vi "ziOpen.vi"(3 "Error In":errorcluster, 4 "Port obsolete (auto)":u16, 5 "Hostname obsolete (auto)":string, 6 "Address":string="DEV") -> (0 "Error Out":errorcluster, 1 "Selected Device":string, 2 "HandleOut":T1 {"Handle" format="0x%08x"; "Conn" format="0x%08x"})   [LabVIEW 2019, in "Zurich Instruments LabOne.lvlib"]
doc: "Creates a connection to a Data Server. <b>Address</b> is of the format {<host>}{:<port}{::<Device ID>}. Usually it is sufficient to provide the <b>Device ID</b> only. The host and port are then determined by network discovery. Should the discovery not work, prepend <host>:<port>:: to the Device ID. Examples are \"myhf2.company.com:8004::dev466\" or \"myhf2.company.com:8004\". In the latter case the first found instrument on the data server listening on myhf2.company.com:8004 will be selected."
uses:
  Zurich Instruments LabOne.lvlib
  ziTypeHandle.ctl
  ziTypeDisovery.ctl
  Private/ziLV64.dll
panel:
  out "auto-connected":bool
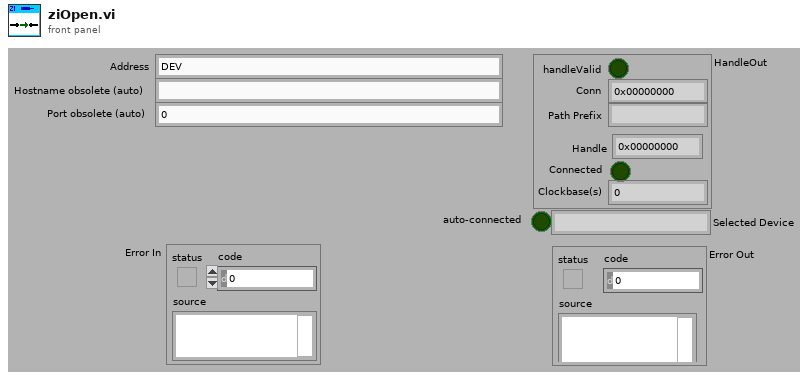
[diagram p1: front panel]
types:
  T1 = typedef "Zurich Instruments LabOne.lvlib/ziTypeHandle.ctl" = cluster{"handleValid":bool, "Conn":u64, "Path Prefix":string, "Handle":u64, "Connected":bool, "Clockbase(s)":dbl}
  T2 = typedef "Zurich Instruments LabOne.lvlib/ziTypeDisovery.ctl" = cluster{"timestamp":u64, "deviceid":string, "devicetype":string, "serveraddress":string, "serverport":u32, "apilevel":u32, "discoverable":bool, "interface":string, "connected":string, "available":bool, "owner":string, "status":string, "options ":string, "serverversion":string}
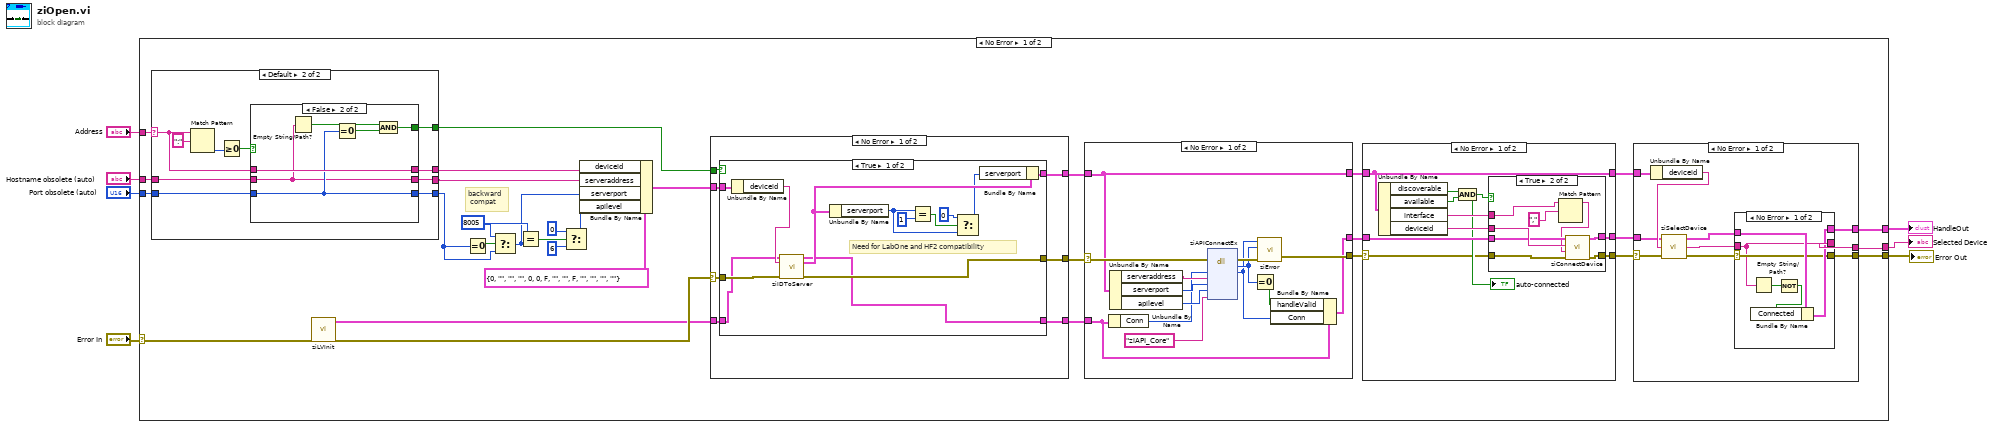
[diagram p0: block diagram]
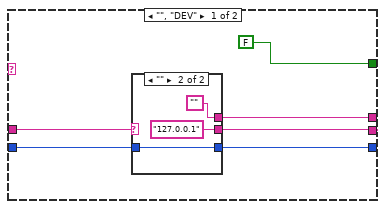
[diagram p2: hidden frame]
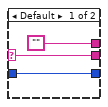
[diagram p3: hidden frame]
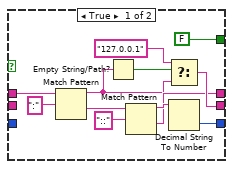
[diagram p4: hidden frame]
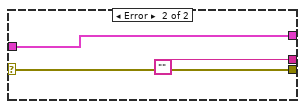
[diagram p6: hidden frame]
diagram:
  n1 = case shown="No Error" "Error In" {
    selector: "Error In" -> [w10 w167]
    tunnel: [w38 w167] -> w7
    tunnel: [w37 _] -> w6
    tunnel: "Hostname obsolete (auto)" -> [w30 _]
    tunnel: "Port obsolete (auto)" -> [w31 _]
    tunnel: [w36 _] -> w5
    tunnel: "Address" -> [w29 _]
    frame No Error {
      w16 = u32 8005
      # "backward\n compat"
      n2 = case shown="Default" w29 {
        selector: w29 -> [_ w53]
        tunnel: w30 -> [w44 w59]
        tunnel: w31 -> [w43 w55]
        tunnel: [w42 w60] -> w17
        tunnel: [w41 w58] -> w23
        tunnel: [w40 w57] -> w22
        tunnel: [FALSE w56] -> w19
        frame "", "DEV" {
          n3 = case shown="\"\"" w44 {
            selector: w44 -> [w46 _]
            tunnel: w43 -> [w45 w50]
            tunnel: [w45 w50] -> w42
            tunnel: [w46 "127.0.0.1"] -> w41
            tunnel: ["" ""] -> w40
            frame Default {
            }
            frame "" {
            }
          }
        }
        frame Default {
          n4 = Match Pattern(string=w53, regular expression=":") -> (offset past match=w54:i32)  [unwired: 1 in, 3 out]
          n5 = Greater Or Equal To 0?(x=w54) -> (x >= 0?=w51:bool)
          n6 = case shown="False" w51 {
            tunnel: [w65 w77] -> w60
            tunnel: w59 -> [_ w74]
            tunnel: [w67 w74] -> w58
            tunnel: w53 -> [w71 w78]
            tunnel: [w64 w78] -> w57
            tunnel: [FALSE w75] -> w56
            tunnel: w55 -> [_ w77]
            frame True {
              n7 = Match Pattern(string=w71, regular expression=":") -> (before substring=w62:string, after substring=w68:string)  [unwired: 1 in, 2 out]
              n8 = Empty String/Path?(string/path=w62) -> (empty?=w61:bool)
              n9 = Match Pattern(string=w68, regular expression="::") -> (before substring=w66:string, after substring=w64:string)  [unwired: 1 in, 2 out]
              n10 = Select(t="127.0.0.1", s=w61, f=w62) -> (s? t:f=w67:string)
              n11 = Decimal String To Number(string=w66) -> (number=w65:i32)  [unwired: 2 in, 1 out]
            }
            frame False {
              n12 = Empty String/Path?(string/path=w74) -> (empty?=w73:bool)
              n13 = Equal To 0?(x=w77) -> (x = 0?=w76:bool)
              n14 = And(x=w73, y=w76) -> (x .and. y?=w75:bool)
            }
          }
        }
      }
      n15 = call "ziLVInit.vi"("Error In"=w10) -> ("Error Out"=w9:errorcluster, "ziHandle"=w8:T1)  [unwired: 9 in]
      n16 = Equal To 0?(x=w17) -> (x = 0?=w18:bool)
      n17 = Select(t=w16, s=w18, f=w17) -> (s? t:f=w11:u32)
      n18 = Equal?(x=w16, y=w11) -> (x = y?=w15:bool)
      n19 = Select(t=u32 0, s=w15, f=u32 6) -> (s? t:f=w12:u32)
      n20 = Bundle By Name(cluster=T2 {"timestamp"=0, "deviceid"="", "devicetype"="", "serveraddress"="", "serverport"=0, "apilevel"=0, "discoverable"=FALSE, "interface"="", "connected"="", "available"=FALSE, "owner"="", "status"="", "options "="", "serverversion"=""} ("ziDiscovery"), "deviceid"=w22, "serveraddress"=w23, "serverport"=w11, "apilevel"=w12) -> (w25:T2)
      n21 = case shown="No Error" w9 {
        selector: w9 -> [w130 w149]
        tunnel: [w129 w149] -> w32
        tunnel: [w128 w147] -> w28
        tunnel: w19 -> [w127 _]
        tunnel: w25 -> [w126 w147]
        tunnel: w8 -> [w125 w148]
        tunnel: [w124 w148] -> w21
        frame No Error {
          n22 = case shown="True" w127 {
            tunnel: w130 -> [w143 w146]
            tunnel: [w142 w146] -> w129
            tunnel: [w140 w145] -> w128
            tunnel: w126 -> [w134 w145]
            tunnel: w125 -> [w131 w144]
            tunnel: [w132 w144] -> w124
            frame True {
              # "Need for LabOne and HF2 compatibility"
              n23 = Unbundle By Name(w134) -> ("deviceid"=w133:string)
              n24 = call "ziIDToServer.vi"("ziHandle In"=w131, "Device ID"=w133, "Error In"=w143) -> ("ziHandle Out"=w132:T1, "ziDiscovery"=w141:T2, "Error Out"=w142:errorcluster)  [unwired: 10 in]
              n25 = Unbundle By Name(w141) -> ("serverport"=w136:u32)
              n26 = Equal?(x=w136, y=u32 1) -> (x = y?=w138:bool)
              n27 = Select(t=u32 0, s=w138, f=w136) -> (s? t:f=w135:u32)
              n28 = Bundle By Name(cluster=w141, "serverport"=w135) -> (w140:T2)
            }
            frame False {
            }
          }
        }
        frame Error {
        }
      }
      n29 = case shown="No Error" w32 {
        selector: w32 -> [w159 w166]
        tunnel: [w162 w166] -> w33
        tunnel: w28 -> [w156 w165]
        tunnel: [w156 w165] -> w27
        tunnel: w21 -> [w152 w164]
        tunnel: [w151 w164] -> w20
        frame No Error {
          n30 = Unbundle By Name(w152) -> ("Conn"=w154:u64)
          n31 = Unbundle By Name(w156) -> ("serveraddress"=w158:string, "serverport"=w157:u32, "apilevel"=w155:u32)
          n32 = dll-call lib="G:/01_software/CryoTUM/sub_vi-s/Equipment/Zurich Instruments LabOne/Private/ziLV*.*" fn="ziAPIConnectEx"(error in=w159, "Conn"=w154, "hostname"=w158, "Port"=w157, "ZIAPIVersion_enum"=w155, "Implementation"="ziAPI_Core") -> (error out=w163:errorcluster, "return type"=w161:u32, "Conn"=w153:u64)  [unwired: 6 in, 1 out]
          n33 = Equal To 0?(x=w161) -> (x = 0?=w150:bool)
          n34 = call "ziError.vi"("Conn"=w153, "ziErrorCode"=w161, "Error In"=w163) -> ("Error Out"=w162:errorcluster)  [unwired: 3 in]
          n35 = Bundle By Name(cluster=w152, "handleValid"=w150, "Conn"=w153) -> (w151:T1)
        }
        frame Error {
        }
      }
      n36 = case shown="No Error" w33 {
        selector: w33 -> [w101 w122]
        tunnel: w27 -> [w102 w121]
        tunnel: w20 -> [w109 w123]
        tunnel: [w108 w123] -> w35
        tunnel: [w107 w122] -> w34
        tunnel: [w102 w121] -> w26
        frame No Error {
          n37 = Unbundle By Name(w102) -> ("discoverable"=w104:bool, "available"=w105:bool, "interface"=w106:string, "deviceid"=w110:string)
          n38 = And(x=w104, y=w105) -> (x .and. y?=w103:bool)
          "auto-connected" <- w103
          n39 = case shown="True" w103 {
            tunnel: w110 -> [_ w120]
            tunnel: w109 -> [w111 w116]
            tunnel: [w111 w119] -> w108
            tunnel: [w112 w118] -> w107
            tunnel: w106 -> [_ w113]
            tunnel: w101 -> [w112 w117]
            frame False {
            }
            frame True {
              n40 = Match Pattern(string=w113, regular expression="," ("replace string (\"\")")) -> (before substring=w115:string)  [unwired: 1 in, 3 out]
              n41 = call "ziConnectDevice.vi"("Error In"=w117, "Device Interface"=w115, "Device Serial"=w120, "Handle In"=w116) -> ("Error Out"=w118:errorcluster, "Handle Out"=w119:T1)  [unwired: 6 in]
            }
          }
        }
        frame Error {
        }
      }
      n42 = case shown="No Error" w34 {
        selector: w34 -> [w88 w98]
        tunnel: [w79 w98] -> w38
        tunnel: w35 -> [w85 w100]
        tunnel: [w82 w100] -> w37
        tunnel: [w80 ""] -> w36
        tunnel: w26 -> [w87 _]
        frame No Error {
          n43 = Unbundle By Name(w87) -> ("deviceid"=w86:string)
          n44 = call "ziSelectDevice.vi"("Error In"=w88, "Device (first)"=w86, "Handle In"=w85) -> ("Error Out"=w84:errorcluster, "Selected Device"=w81:string, "Handle Out"=w83:T1)
          n45 = case shown="No Error" w84 {
            selector: w84 -> [w92 w95]
            tunnel: w83 -> [w94 w97]
            tunnel: w81 -> [w91 w96]
            tunnel: [w93 w97] -> w82
            tunnel: [w91 w96] -> w80
            tunnel: [w92 w95] -> w79
            frame No Error {
              n46 = Empty String/Path?(string/path=w91) -> (empty?=w90:bool)
              n47 = Not(x=w90) -> (.not. x?=w89:bool)
              n48 = Bundle By Name(cluster=w94, "Connected"=w89) -> (w93:T1)
            }
            frame Error {
            }
          }
        }
        frame Error {
        }
      }
    }
    frame Error {
    }
  }
  "Error Out" <- w7
  "HandleOut" <- w6
  "Selected Device" <- w5
